vi "DUTResults.vi"(9 "Left Coordinate":i16, 10 "Top Coordinate":i16, 11 "Sequence Context In":refnum<k7>) -> (0 "error out":errorcluster)   [LabVIEW 2021]
doc: "Calls TesStand API to display test result banners."
uses:
  <vilib>/addons/TestStand/_TSUtility.llb/TestStand - Get Property Value (String).vi
  <vilib>/addons/TestStand/_TSUtility.llb/TestStand - Get Property Value (Number {Unsigned 32-bit Integer}).vi
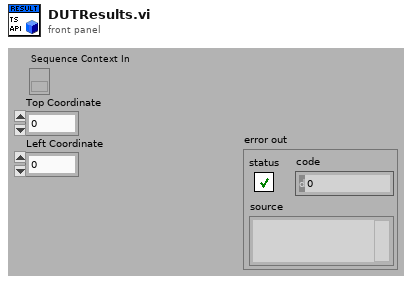
[diagram p1: front panel]
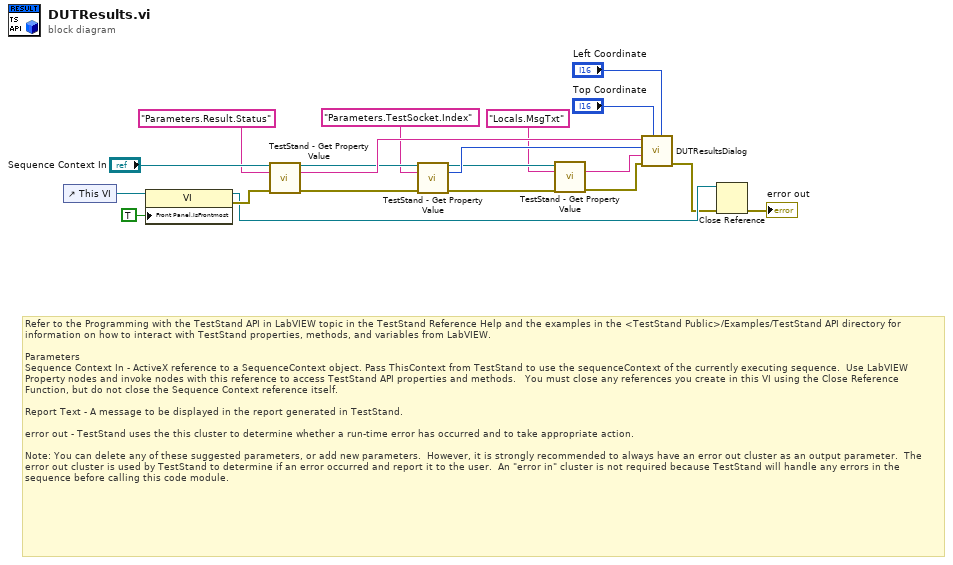
[diagram p0: block diagram]
diagram:
  # "Refer to the Programming with the TestStand API in LabVIEW topic in the TestStand Reference Help and the examples in the <TestStand Public>/Examples/TestStand API directory for information on how to interact with TestStand properties, methods, and variables from LabVIEW.\n\nParameters\nSequence Context In - ActiveX reference to a SequenceContext object. Pass ThisContext from TestStand to use the sequenceContext of the currently executing sequence.  Use LabVIEW Property nodes and invoke nodes with this reference to access TestStand API properties and methods.   You must close any references you create in this VI using the Close Reference Function, but do not close the Sequence Context reference itself.\n\nReport Text - A message to be displayed in the report generated in TestStand. \n\nerror out - TestStand uses the this cluster to determine whether a run-time error has occurred and to take appropriate action.  \n\nNote: You can delete any of these suggested parameters, or add new parameters.  However, it is strongly recommended to always have an error out cluster as an output parameter.  The error out cluster is used by TestStand to determine if an error occurred and report it to the user.  An \"error in\" cluster is not required because TestStand will handle any errors in the sequence before calling this code module."
  n1 = control-ref of="This VI"() -> (w6:refnum<vi>)
  n2 = property class="VI"(reference=w6, "Front Panel.IsFrontmost"=TRUE ("Front Panel Window:Is Frontmost")) -> (reference out=w3:refnum<vi>, error out=w4:errorcluster)  [unwired: 1 in]
  n3 = call-poly <vilib>:"TestStand - Get Property Value.vi"("Sequence Context In"="Sequence Context In", "Lookup String"="Parameters.Result.Status", "error in (no error)"=w4) -> ("Sequence Context Out"=w17:refnum<k7>, "Value"=w18:string, "error out"=w16:errorcluster)  [unwired: 10 in]
  n4 = call-poly <vilib>:"TestStand - Get Property Value.vi"("Sequence Context In"=w17, "Lookup String"="Parameters.TestSocket.Index", "error in (no error)"=w16) -> ("Sequence Context Out"=w13:refnum<k7>, "Value"=w14:u32, "error out"=w12:errorcluster)  [unwired: 10 in]
  n5 = call-poly <vilib>:"TestStand - Get Property Value.vi"("Sequence Context In"=w13, "Lookup String"="Locals.MsgTxt", "error in (no error)"=w12) -> ("Value"=w10:string, "error out"=w9:errorcluster)  [unwired: 10 in, 1 out]
  n6 = call "DUTResultsDialog.vi"("Left Coordinate"="Left Coordinate", "Top Coordinate"="Top Coordinate", "error in (no error)"=w9, "MessageTxt"=w10, "TestSocketIndex"=w14, "Value"=w18) -> ("error out"=w2:errorcluster)  [unwired: 5 in]
  n7 = Close Reference(reference=w3, error in (no error)=w2) -> (error out=→"error out":errorcluster)
